vi "腐蚀膨胀.vi"() -> ()   [LabVIEW 2018]
uses:
  <vilib>/vision/NI_Vision_Development_Module.lvlib
panel:
  in  "Structuring Element":i32[][](array[numeric])=[[1, 1, 1], [1, 1, 1], [1, 1, 1]]
  in  "Operation":T1(ring)=enum."Erode"
  out "Image 2":T2(plugin-control)
  out "Image":T2(plugin-control)
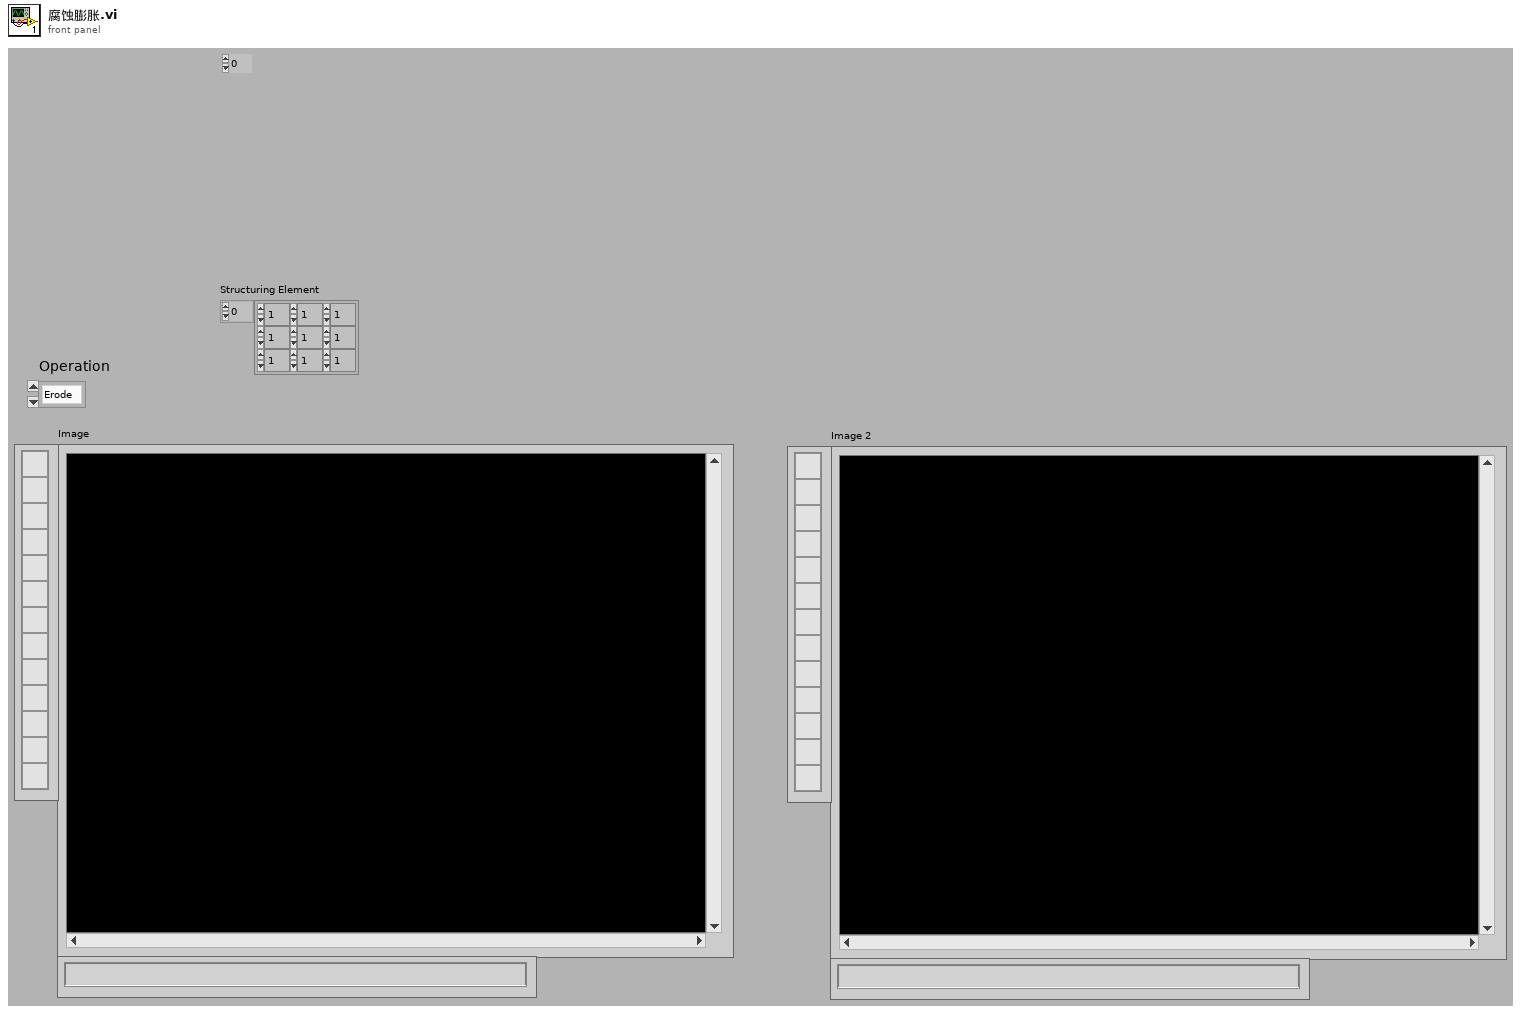
[diagram p1: front panel]
types:
  T1 = enum32{"AutoM", "Close", "Dilate", "Erode", "Gradient", "Gradient in", "Gradient out", "HitMiss", "Open", "PClose", "POpen", "Thick", "Thin"}
  T2 = typedef "IMAQ Image.ctl" = refnum<image>
  T3 = typedef "Image Type" = u32
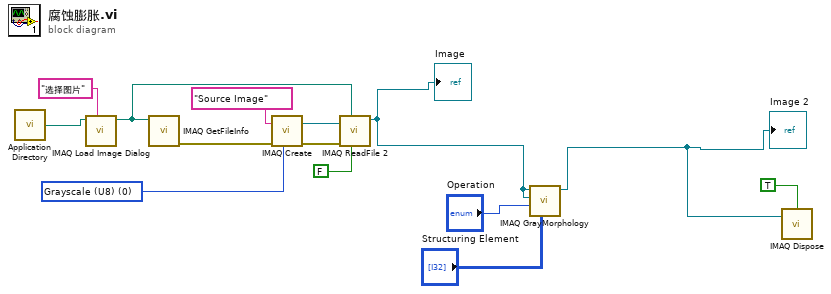
[diagram p0: block diagram]
diagram:
  w7 = T3 0 items=["Grayscale (U8)", "Grayscale (I16)", "Grayscale (SGL)", "Complex (CSG)", "RGB (U32)", "HSL (U32)", "RGB (U64)", "Grayscale (U16)"] ("Image Type")
  n1 = call <vilib>:"Application Directory.vi"() -> ("Application Directory"=w8:path)
  n2 = call "IMAQ Load Image Dialog"("Prompt"="选择图片" ("prompt"), "Start Path"=w8) -> ("Path"=w14:path)  [unwired: 7 in, 2 out]
  n3 = call "IMAQ GetFileInfo"("File Path"=w14) -> ("error out"=w12:errorcluster)  [unwired: 4 in, 6 out]
  n4 = call "IMAQ Create"("Image Name"="Source Image", "Image Type"=w7, "error in (no error)"=w12) -> ("New Image"=w10:T2, "error out"=w9:errorcluster)  [unwired: 2 in]
  n5 = call "IMAQ ReadFile 2"("Use File Path Image Type"=FALSE, "File Path"=w14, "error in (no error)"=w9, "Image"=w10) -> ("Image Out"=w4:T2)  [unwired: 3 in, 4 out]
  "Image" <- w4
  n6 = call "IMAQ GrayMorphology"("Structuring Element"="Structuring Element", "Operation"="Operation", "Image Dst"=w4, "Image Src"=w4) -> ("Image Dst Out"=w3:T2)  [unwired: 6 in, 1 out]
  "Image 2" <- w3
  n7 = call "IMAQ Dispose"("All Images? (No)"=TRUE, "Image"=w3) -> ()  [unwired: 1 in, 4 out]
